vi "collectLT_res_v1.vi"(2 "stream?":bool, 3 "data file":path=path "C:/Users/Labmember/Desktop/Data/temp" caption="data dir.") -> (0 "cts/sec":dbl, 1 "total counts":i32)   [LabVIEW 2015]
uses:
  phlib.dll
panel:
  out "acq time":i32
  out "Fifo overrun":bool
  out "buffer size":i32
  out "exp iterations":i32=5
  out "counts per\niteration":i32[](array[numeric])
  out "trunc buffer":u32[](array[numeric]) format="%08x"
  out "buffer":u32[](array[numeric]) format="%08x"
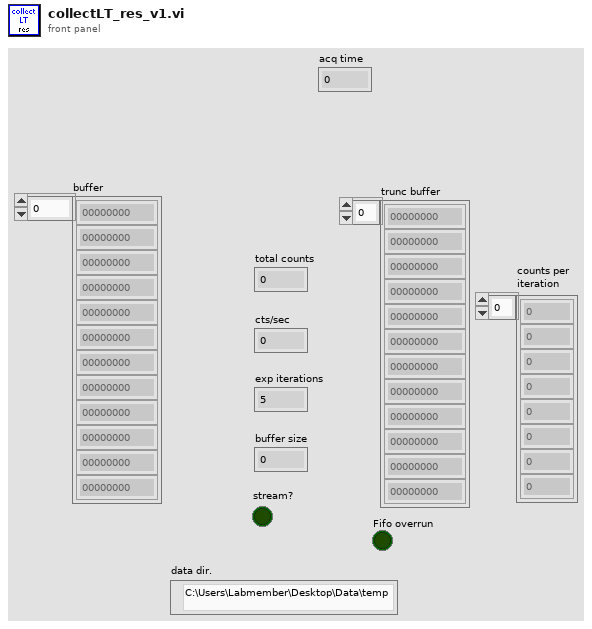
[diagram p1: front panel]
types:
  T1 = enum16{"open", "replace", "create", "open or create", "replace or create", "replace or create with confirmation"}
  T2 = typedef "LVRectTypeDef.ctl" = cluster{"Left":i16, "Top":i16, "Right":i16, "Bottom":i16}
  T3 = cluster{"Xpixels":i32, "Vxminref":dbl, "Vxmaxref":dbl, "P":dbl, "Ypixels":i32, "Vyminref":dbl, "Vymaxref":dbl, "srate":sgl, "sAOxy":i32, "timeout":dbl, "type":string, "date":string, "time":string, "Colormap":u16, "Drawing Mode":u16, "Scanning Mode":u16, "square pixels":bool, "square matrix":bool, "Xpixels Img":i32, "Vx-min Img":dbl, "VX-max Img":dbl, "Ypixels Img":i32, "Vy-min Img":dbl, "Vy-max Img ":dbl, "Angle Img":dbl, "autoshutter":bool, "finite":bool, "cont":bool, "wavdet":bool, "measpoints":i32, "avpp":i32, "bufferAO":i32, "bufferAI":i32, "starttick":u32, "waveform":path, "Vx-ref":dbl, "Vy-ref":dbl, "refreshrate":dbl, "refreshbuffer":i32, "tt_cycles":i32, "motorref":refnum<k7>, "mirrorswitch":refnum<k7>, "sample mode":i32, "maxbufferAI":i32, "srateAODO":sgl, "bin":sgl, "Pel":sgl, "Angle draw":dbl, "srate Img":sgl, "ROIimg_plotbounds":T2, "auto OD":bool, "ODfilt":u16, "aAI":i32[], "aCI":i32[], "aAO":u32[], "aDO":u32[], "refwfsize":dbl, "Lifetime":bool, "Vz-Img":dbl, "Vz-ref":dbl, "Vz-reset":dbl, "AIoverride":bool, "aAS":u32[], "XYZstart":dbl[]}
  T4 = cluster{"initialized":bool, "devidx":i32, "Ch0 Level":i32, "Ch0 ZeroX":i32, "Ch1 Level":i32, "Ch1 ZeroX":i32, "sync rate":i32, "resolution":i32, "acq time":i32, "acq rate":i32, "# bins":u32, "Bin size":enum16{"1", "2", "4", "8", "16", "32", "64", "128"}, "min photons":u32, "truncate":u32}
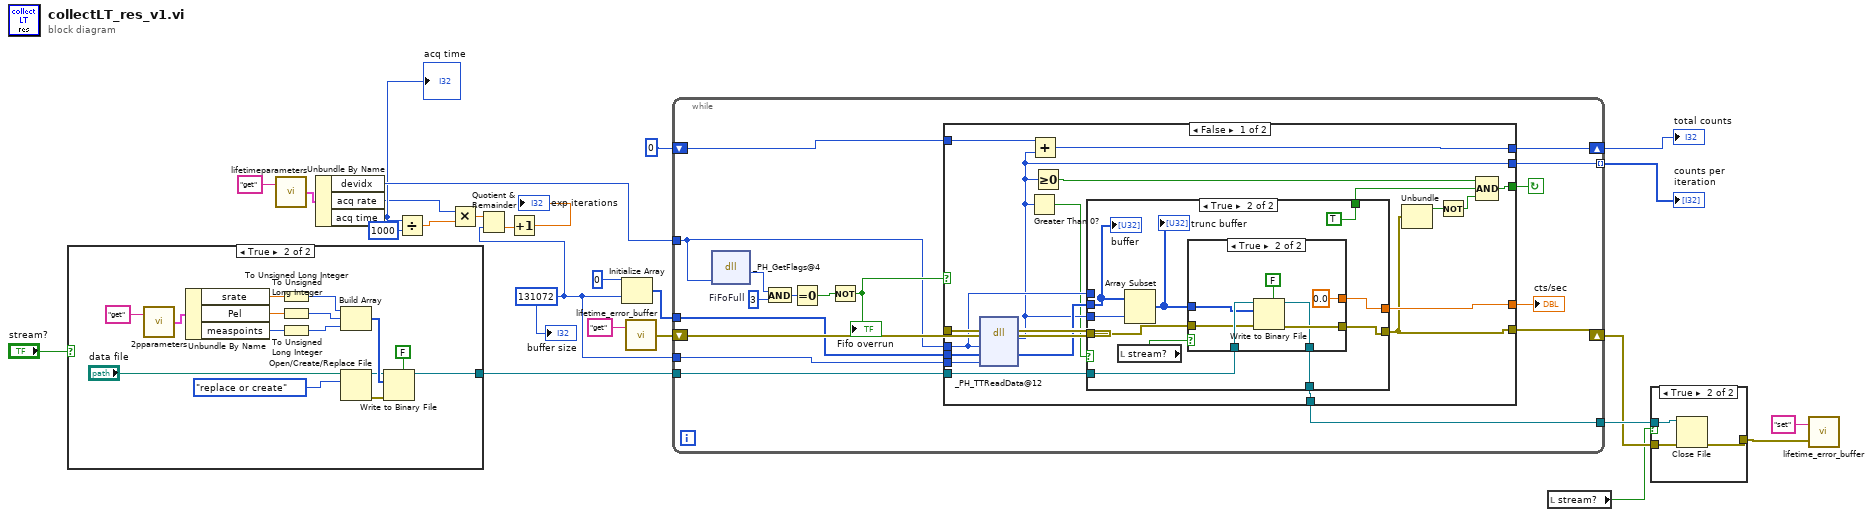
[diagram p0: block diagram]
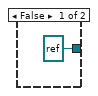
[diagram p3: hidden frame]
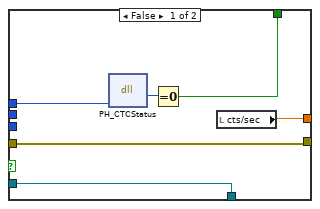
[diagram p4: hidden frame]
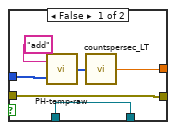
[diagram p5: hidden frame]
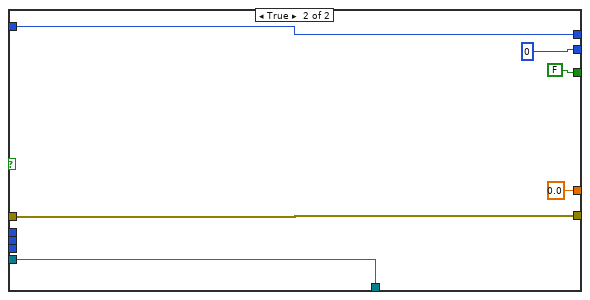
[diagram p6: hidden frame]
diagram:
  w11 = 131072 ("y")
  n1 = case shown="True" "stream?" {
    tunnel: [refnum<file> refnum ("refnum out") w29] -> w7
    frame False {
    }
    frame True {
      n2 = call "2pparameters.vi"("command"="get") -> ("params out"=w39:T3)  [unwired: 1 in]
      n3 = Unbundle By Name(w39) -> ("srate"=w37:sgl, "Pel"=w36:sgl, "measpoints"=w34:i32)
      n4 = To Unsigned Long Integer(number=w37) -> (unsigned 32bit integer=w38:u32)
      n5 = To Unsigned Long Integer(number=w36) -> (unsigned 32bit integer=w35:u32)
      n6 = To Unsigned Long Integer(number=w34) -> (unsigned 32bit integer=w33:u32)
      n7 = Build Array(w38, w35, w33) -> (w32:u32[])
      n8 = Open/Create/Replace File(file path (use dialog)="data file", operation (0:open)=T1."replace or create") -> (refnum out=w31:refnum<file>, error out=w30:errorcluster)  [unwired: 4 in, 1 out]
      n9 = Write to Binary File(file (use dialog)=w31, data=w32, error in=w30, 5:FALSE ("prepend array or string size? (T)")) -> (refnum out=w29:refnum<file>)  [unwired: 2 in, 2 out]
    }
  }
  n10 = call "lifetimeparameters.vi"("command"="get") -> ("Params out"=w22:T4)  [unwired: 1 in]
  n11 = Unbundle By Name(w22) -> ("devidx"=w21:i32, "acq rate"=w12:i32, "acq time"=w13:i32)
  "acq time" <- w13
  n12 = Divide(x=w13, y=1000) -> (x/y=w1:dbl)
  n13 = Multiply(x=w12, y=w1) -> (x*y=w10:dbl)
  n14 = Quotient & Remainder(x=w10, y=w11) -> (floor(x/y)=w14:dbl)  [unwired: 1 out]
  n15 = Increment(x=w14) -> (x+1=→"exp iterations":dbl)
  n16 = Initialize Array(u32 0, w11) -> (w17:u32[])
  n17 = call "lifetime_error_buffer.vi"("command"="get") -> ("error out"=w24:errorcluster)  [unwired: 1 in]
  n18 = while {
    tunnel: w21 -> [w44]
    shift-right: [w57] -> w5
    shift-left: w24 -> [w58]
    tunnel: [w54] -> w19 mode=indexing
    tunnel: w17 -> [w56]
    tunnel: w11 -> [w55]
    shift-right: [w53] -> w16
    shift-left: 0 ("return type") -> [w52]
    tunnel: w7 -> [w43]
    tunnel: [w42] -> w6
    stop <- w46 continue-if-true
    w48 = 3  # FiFoFull
    n19 = dll-call lib="phlib.dll" fn="_PH_GetFlags@4" label="PH_GetFlags"("devidx"=w44) -> (w50:i32)  [unwired: 4 in, 2 out]
    n20 = And(x=w50, y=w48) -> (x .and. y?=w49:i32)
    n21 = Equal To 0?(x=w49) -> (x = 0?=w51:bool)
    n22 = Not ("CTCDone")(x=w51) -> (.not. x?=w47:bool)
    "Fifo overrun" <- w47
    n23 = case shown="False" w47 {
      tunnel: w58 -> [w77 w110]
      tunnel: [w66 w110] -> w57
      tunnel: w44 -> [w71 _]
      tunnel: w56 -> [w76 _]
      tunnel: w55 -> [w75 _]
      tunnel: [w60 0 ("return type")] -> w54
      tunnel: [w74 w109] -> w53
      tunnel: w52 -> [w73 w109]
      tunnel: [w61 FALSE] -> w46
      tunnel: [w69 0.0 ("Avg cts/s")] -> w45
      tunnel: w43 -> [w68 w107]
      tunnel: [w67 w107] -> w42
      frame False {
        n24 = dll-call lib="phlib.dll" fn="_PH_TTReadData@12" label="PH_TTReadData"(error in=w77, "devidx"=w71, "buffer"=w76, "blocksize"=w75) -> (error out=w72:errorcluster, "return type"=w60:i32, "buffer"=w70:u32[])  [unwired: 4 in, 1 out]
        n25 = Greater Than 0?(x=w60) -> (x > 0?=w59:bool)
        n26 = Add(x=w73, y=w60) -> (x+y=w74:i32)
        n27 = Greater Or Equal To 0?(x=w60) -> (x >= 0?=w62:bool)
        n28 = case shown="True" w59 {
          tunnel: [w83 w86] -> w66
          tunnel: w72 -> [w83 w87]
          tunnel: [w81 TRUE] -> w63
          tunnel: w71 -> [w80 _]
          tunnel: w70 -> [_ w92]
          tunnel: w60 -> [_ w91]
          tunnel: [w79 w90] -> w69
          tunnel: w68 -> [w78 w88]
          tunnel: [w78 w84] -> w67
          frame False {
            n29 = dll-call lib="phlib.dll" fn="PH_CTCStatus"("devidx"=w80) -> (w82:i32)  [unwired: 4 in, 2 out]
            n30 = Equal To 0?(x=w82) -> (x = 0?=w81:bool)
            n31 = local read "cts/sec"() -> (w79:dbl)
          }
          frame True {
            n32 = local read "stream?"() -> (w85:bool)
            n33 = Array Subset(array=w92, length=w91) -> (w93:u32[])  [unwired: 1 in]
            "trunc buffer" <- w93
            n34 = case shown="True" w85 {
              tunnel: w93 -> [w98 w103]
              tunnel: [w96 0.0 ("Avg cts/s")] -> w90
              tunnel: w88 -> [w94 w104]
              tunnel: w87 -> [w95 w102]
              tunnel: [w95 w101] -> w86
              tunnel: [w94 w100] -> w84
              frame False {
                n35 = call "PH-temp-raw.vi"("array in"=w98, "command"="add") -> ("array out"=w99:u32[])
                n36 = call "countspersec_LT.vi"("1D PH data"=w99) -> ("Avg cts/s"=w96:dbl)
              }
              frame True {
                n37 = Write to Binary File(file (use dialog)=w104, data=w103, error in=w102, 5:FALSE ("prepend array or string size? (T)")) -> (refnum out=w100:refnum<file>, error out=w101:errorcluster)  [unwired: 2 in, 1 out]
              }
            }
            "buffer" <- w92
          }
        }
        n38 = Unbundle(w66) -> ("status"=w65:bool)  [unwired: 2 out]
        n39 = Not(x=w65) -> (.not. x?=w64:bool)
        n40 = Compound Arithmetic op=AND(w62, w63, w64) -> (w61:bool)
      }
      frame True {
      }
    }
    "cts/sec" <- w45
  }
  "counts per\niteration" <- w19
  "total counts" <- w16
  n41 = local read "stream?"() -> (w3:bool)
  n42 = case shown="True" w3 {
    tunnel: w6 -> [_ w116]
    tunnel: w5 -> [w113 w115]
    tunnel: [w113 w114] -> w4
    frame False {
    }
    frame True {
      n43 = Close File(refnum=w116, error in=w115) -> (error out=w114:errorcluster)  [unwired: 1 out]
    }
  }
  n44 = call "lifetime_error_buffer.vi"("error in"=w4, "command"="set") -> ()  [unwired: 1 out]
  "buffer size" <- w11
